vi "OhmConfig.vi"(8 "error in (no error)":errorcluster, 10 "Function (0: Volts)":u16(ring) items=["AUTO", "2", "2O", "200", "2k", "20k", "200k", "2M", "20M", "200M"], 11 "VISA resource name":refnum<visa-resource-name>) -> (0 "error out":errorcluster, 3 "VISA resource name out":refnum<visa-resource-name>)   [LabVIEW 2016]
uses:
  <instrlib>/Keithley 24XX/Keithley 24XX.lvlib
panel:
  out "concatenated string":string
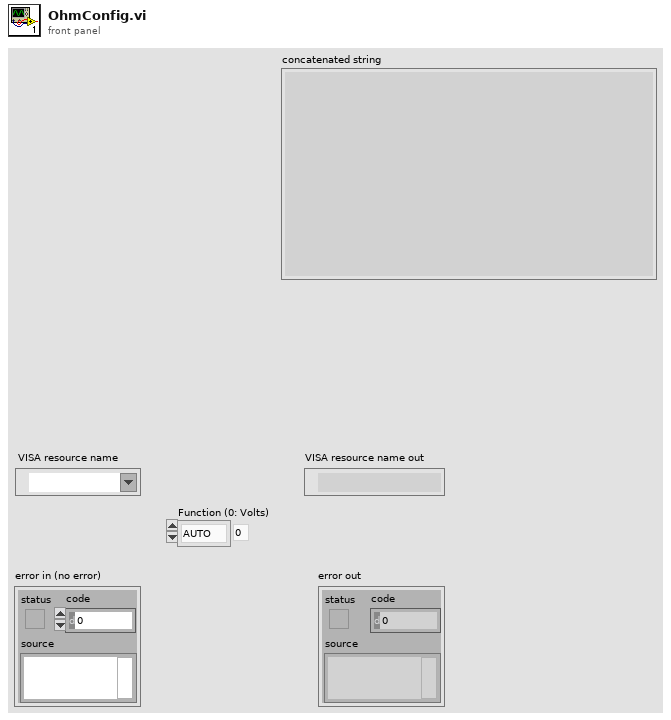
[diagram p1: front panel]
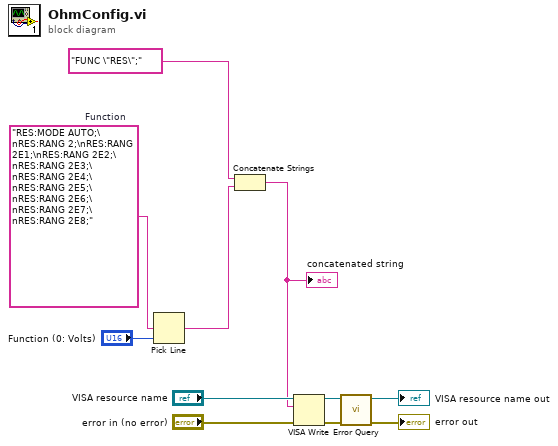
[diagram p0: block diagram]
diagram:
  w5 = "RES:MODE AUTO;\nRES:RANG 2;\nRES:RANG 2E1;\nRES:RANG 2E2;\nRES:RANG 2E3;\nRES:RANG 2E4;\nRES:RANG 2E5;\nRES:RANG 2E6;\nRES:RANG 2E7;\nRES:RANG 2E8;"  # Function
  n1 = Pick Line(multi-line string=w5, line index="Function (0: Volts)") -> (output string=w2:string)  [unwired: 1 in]
  n2 = Concatenate Strings("FUNC \"RES\";", w2) -> (w1:string)
  "concatenated string" <- w1
  n3 = VISA Write(VISA resource name="VISA resource name", write buffer=w1, error in (no error)="error in (no error)") -> (VISA resource name out=w7:refnum<visa-resource-name>, error out=w6:errorcluster)  [unwired: 1 out]
  n4 = call <instrlib>:"Error Query.vi"("error in (no error)"=w6, "VISA resource name"=w7) -> ("error out"=→"error out":errorcluster, "VISA resource name out"=→"VISA resource name out":refnum<visa-resource-name>)  [unwired: 6 in, 2 out]
